vi "Datasheet Find Channel by SN Yield.vi"(7 "Model Number":string, 8 "error in (no error)":errorcluster, 11 "Data":T1) -> (0 "error out":errorcluster, 3 "Sample Results":T8)   [LabVIEW 2011]
uses:
  CGI Yield Results.ctl
  TDMS/TDMS Serial Number.ctl
  TDMS/TDMS File.ctl
  TDMS/TDMS Run.ctl
  TDMS/TDMS Channel (Sxx).ctl
  database/Fields/Field Record.ctl
  database/Fields/Field DataTypes.ctl
  database/Fields/Field NextItem.ctl
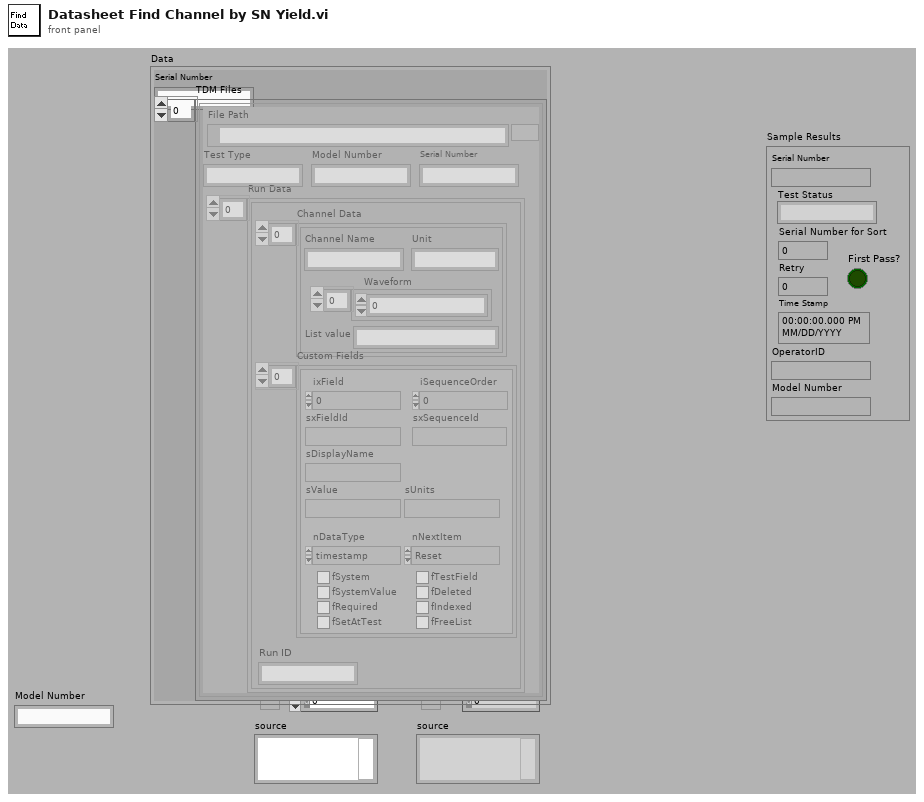
[diagram p1: front panel]
types:
  T1 = typedef "TDMS Serial Number.ctl" = cluster{"Serial Number":string, "TDM Files":T2[]}
  T2 = typedef "TDMS File.ctl" = cluster{"File Path":path, "Run Data":T3[], "Serial Number":string, "Model Number":string, "Test Type":string}
  T3 = typedef "TDMS Run.ctl" = cluster{"Channel Data":T4[], "Custom Fields":T5[], "Run ID":string}
  T4 = typedef "TDMS Channel (Sxx).ctl" = cluster{"Channel Name":string, "Waveform":dbl[], "Unit":string, "List value":string}
  T5 = typedef "Field Record.ctl" = cluster{"ixField":i32, "iSequenceOrder":i32, "sxFieldId":string, "sxSequenceId":string, "sDisplayName":string, "sValue":string, "sUnits":string, "nDataType":T6, "nNextItem":T7, "fSystem":bool, "fSystemValue":bool, "fRequired":bool, "fSetAtTest":bool, "fTestField":bool, "fDeleted":bool, "fIndexed":bool, "fFreeList":bool}
  T6 = typedef "Field DataTypes.ctl" = enum32{"text", "numeric", "list", "timestamp", "boolean"}
  T7 = typedef "Field NextItem.ctl" = enum32{"Reset", "Retain", "Auto-Increment"}
  T8 = typedef "CGI Yield Results.ctl" = cluster{"Model Number":string, "Serial Number for Sort":i32, "Serial Number":string, "Test Status":string, "Time Stamp":timestamp, "OperatorID":string, "Retry":i32, "First Pass?":bool}
  T9 = cluster{"FieldID or Display Name(\"\")":string, "step number":i32}
  T10 = cluster{"FieldID or Display Name(\"\")":string, "step number":i32}[]
  T11 = cluster{"sValue":string, "default value 1":i32}[]
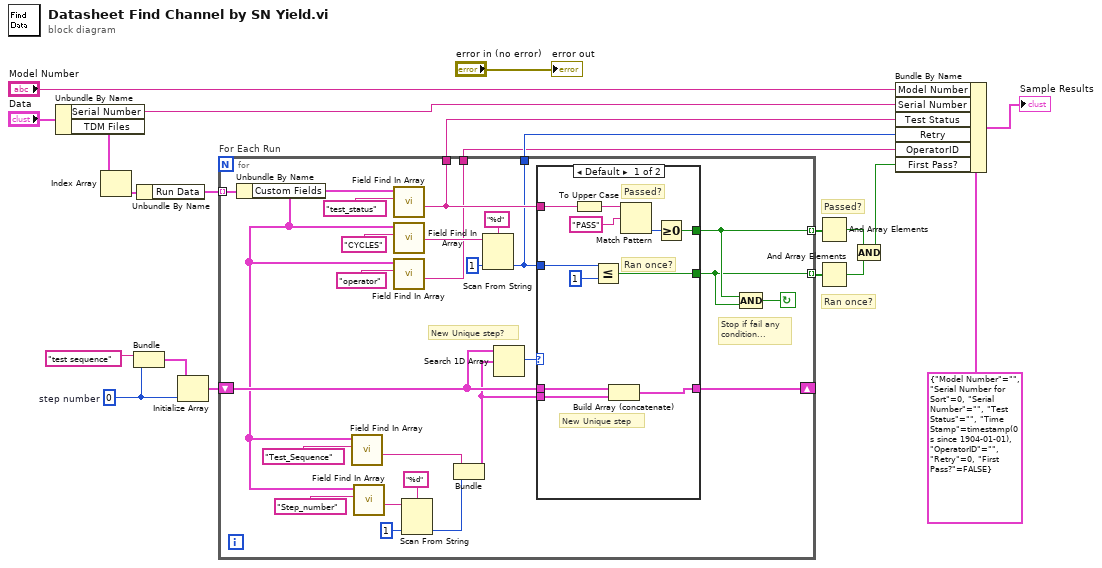
[diagram p0: block diagram]
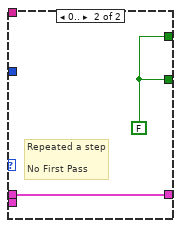
[diagram p2: hidden frame]
diagram:
  w1 = 0  # step number
  # "Ran once?"
  # "Passed?"
  n1 = Unbundle By Name("Data") -> ("Serial Number"=w17:string, "TDM Files"=w13:T2[])
  n2 = Index Array(array=w13) -> (element=w12:T2)  [unwired: 1 in]
  n3 = Bundle("FieldID or Display Name(\"\")"="test sequence" ("FieldID or Display Name(\"\")"), "step number"=w1) -> (w2:T9)  [unwired: 1 out]
  n4 = Unbundle By Name(w12) -> ("Run Data"=w16:T3[])
  n5 = Initialize Array(w2, w1) -> (w15:T10)
  n6 = for "For Each Run" {
    tunnel: w16 -> [w46] mode=indexing
    shift-right: [w31] -> _
    shift-left: w15 -> [w32]
    tunnel: [w38] -> w10 mode=indexing
    tunnel: [w39] -> w11 mode=indexing
    tunnel: [w36] -> w6
    tunnel: [w33] -> w5
    tunnel: [w29] -> w4
    stop <- w37 continue-if-true
    # "Stop if fail any\ncondition..."
    # "New Unique step?"
    n7 = Unbundle By Name(w46) -> ("Custom Fields"=w23:T5[])
    n8 = call "Field Find In Array.vi"("FieldID or Display Name(\"\")"="Test_Sequence" ("FieldID or Display Name(\"\")"), "Field Array"=w23) -> ("sValue"=w24:string)  [unwired: 1 in, 8 out]
    n9 = call "Field Find In Array.vi"("FieldID or Display Name(\"\")"="Step_number" ("FieldID or Display Name(\"\")"), "Field Array"=w23) -> ("sValue"=w42:string)  [unwired: 1 in, 8 out]
    n10 = call "Field Find In Array.vi"("FieldID or Display Name(\"\")"="test_status" ("FieldID or Display Name(\"\")"), "Field Array"=w23) -> ("sValue"=w36:string)  [unwired: 1 in, 8 out]
    n11 = call "Field Find In Array.vi"("FieldID or Display Name(\"\")"="CYCLES" ("FieldID or Display Name(\"\")"), "Field Array"=w23) -> ("sValue"=w35:string)  [unwired: 1 in, 8 out]
    n12 = call "Field Find In Array.vi"("FieldID or Display Name(\"\")"="operator" ("FieldID or Display Name(\"\")"), "Field Array"=w23) -> ("sValue"=w29:string)  [unwired: 1 in, 8 out]
    n13 = Scan From String(format string="%d", input string=w42, default 1=1 ("default value 1")) -> (output 1=w25:i32)  [unwired: 2 in, 3 out]
    n14 = Bundle("sValue"=w24, "default value 1"=w25) -> (w22:cluster{"sValue":string, "default value 1":i32})  [unwired: 1 out]
    n15 = Scan From String(format string="%d", input string=w35, default 1=1 ("default value 1")) -> (output 1=w33:i32)  [unwired: 2 in, 3 out]
    n16 = Search 1D Array(1D array=w32, element=w22) -> (index of element=w40:i32)  [unwired: 1 out]
    n17 = case shown="Default" w40 {
      tunnel: w36 -> [w55 _]
      tunnel: [w56 w59] -> w38
      tunnel: [w51 w59] -> w39
      tunnel: w33 -> [w50 _]
      tunnel: w32 -> [w49 w58]
      tunnel: w22 -> [w48 _]
      tunnel: [w47 w58] -> w31
      frame Default {
        # "Passed?"
        # "Ran once?"
        # "New Unique step"
        n18 = To Upper Case(1:w55) -> (0:w54:string)
        n19 = Less Or Equal?(x=w50, y=1) -> (x <= y?=w56:bool)
        n20 = Build Array (concatenate)(w49, w48) -> (w47:T11)
        n21 = Match Pattern(string=w54, regular expression="PASS" ("format string")) -> (offset past match=w52:i32)  [unwired: 4 out]
        n22 = Greater Or Equal To 0?(x=w52) -> (x >= 0?=w51:bool)
      }
      frame 0.. {
        w59 = FALSE
        # "Repeated a step\n\nNo First Pass"
      }
    }
    n23 = Compound Arithmetic op=AND(w39, w38) -> (w37:bool)
  }
  n24 = And Array Elements(Boolean array=w11) -> (logical AND=w9:bool)
  n25 = And Array Elements(Boolean array=w10) -> (logical AND=w8:bool)
  n26 = Compound Arithmetic op=AND(w9, w8) -> (w7:bool)
  n27 = Bundle By Name(cluster=T8 {"Model Number"="", "Serial Number for Sort"=0, "Serial Number"="", "Test Status"="", "Time Stamp"=timestamp(0 s since 1904-01-01), "OperatorID"="", "Retry"=0, "First Pass?"=FALSE} ("Sample Results"), "Model Number"="Model Number", "Serial Number"=w17, "Test Status"=w6, "Retry"=w5, "OperatorID"=w4, "First Pass?"=w7) -> (→"Sample Results":T8)
  "error out" <- "error in (no error)"
